vi "shutdown.vi"(8 "error in (no error)":errorcluster, 11 "Hamamatsu_C9100-13 in":refnum<class "Hamamatsu_C9100-13.lvclass">) -> (0 "error out":errorcluster, 3 "Hamamatsu_C9100-13 out":refnum<class "Hamamatsu_C9100-13.lvclass">)   [LabVIEW 2013, in "Hamamatsu_C9100-13.lvclass"]
uses:
  Hamamatsu_C9100-13.lvclass
  Camera.lvclass
  Hamamatsu_C9100-13.lvclass/Hamamatsu_C9100-13.ctl
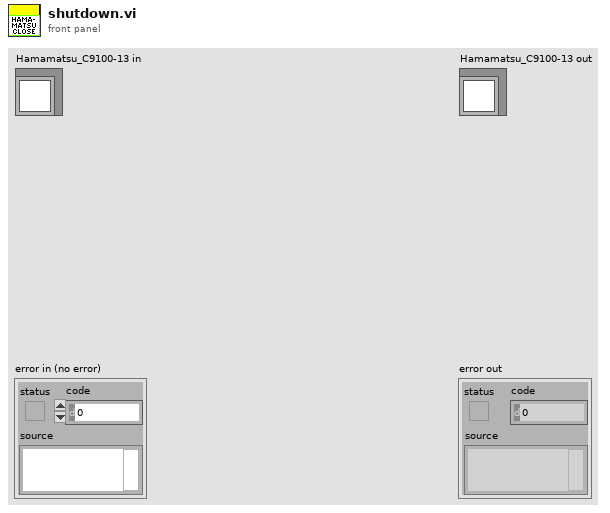
[diagram p1: front panel]
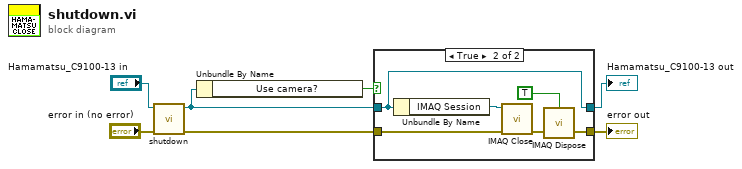
[diagram p0: block diagram]
diagram:
  n1 = call-parent "shutdown.vi"("error in (no error)"="error in (no error)", "Camera in"="Hamamatsu_C9100-13 in") -> ("error out"=w4:errorcluster, "Camera out"=w2:refnum<class "Hamamatsu_C9100-13.lvclass">)  [unwired: 8 in]
  n2 = Unbundle By Name(w2) -> ("Use camera?"=w1:bool)
  n3 = case shown="True" w1 {
    tunnel: w4 -> [w9 w11]
    tunnel: [w9 w13] -> w5
    tunnel: w2 -> [w8 w12]
    tunnel: [w8 w12] -> w3
    frame False {
    }
    frame True {
      n4 = Unbundle By Name(w12) -> ("IMAQ Session"=w10:refnum<k11>)
      n5 = call <vilib>:"IMAQ Close.vi"("error in (no error)"=w11, "IMAQ Session In"=w10) -> ("error out"=w14:errorcluster)  [unwired: 9 in]
      n6 = call "IMAQ Dispose"("All Images? (No)"=TRUE, "error in (no error)"=w14) -> ("error out"=w13:errorcluster)  [unwired: 4 in]
    }
  }
  "error out" <- w5
  "Hamamatsu_C9100-13 out" <- w3
